vi "Control_Create.vi"(0 "reference in":refnum<class "Control.lvclass">, 1 "Object Attributes":T1, 2 "Control Attributes":T3, 5 "error in (no error)":errorcluster) -> (14 "reference out":refnum<class "Control.lvclass">, 19 "error out":errorcluster)   [LabVIEW 2014, in "Control.lvclass"]
uses:
  Control.lvclass
  Attributes.ctl
  Text_class/Text.lvclass
  <vilib>/picture/picture.llb/imagedata.ctl
  Object_class/Attributes.ctl
  Object_class/Coordinates.ctl
  Object_class/Object.lvclass
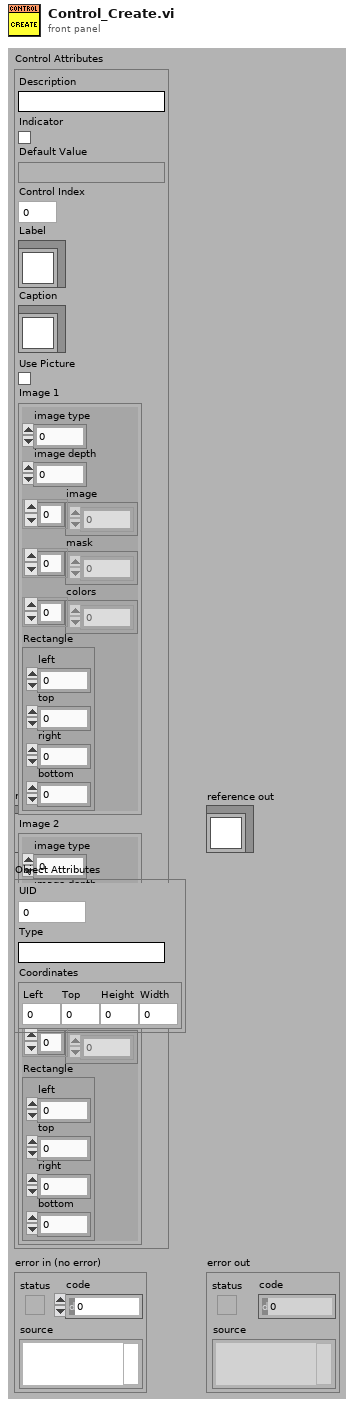
[diagram p1: front panel]
types:
  T1 = typedef "Object.lvclass/Attributes.ctl" = cluster{"UID":i32, "Type":string, "Coordinates":T2}
  T2 = typedef "Object.lvclass/Coordinates.ctl" = cluster{"Left":i32, "Top":i32, "Height":u32, "Width":u32}
  T3 = typedef "Control.lvclass/Attributes.ctl" = cluster{"Description":string, "Indicator":bool, "Default Value":variant, "Control Index":i32, "Label":refnum<class "Text.lvclass">, "Caption":refnum<class "Text.lvclass">, "Use Picture":bool, "Image 1":T4, "Image 2":T4}
  T4 = typedef "imagedata.ctl" = cluster{"image type":i32, "image depth":i32, "image":u8[], "mask":u8[], "colors":u32[], "Rectangle":cluster{"left":i16, "top":i16, "right":i16, "bottom":i16}}
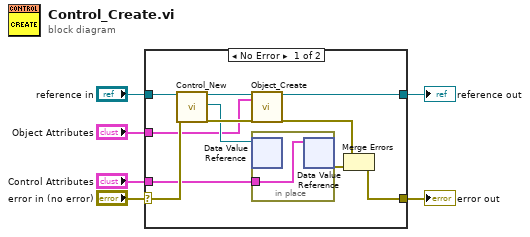
[diagram p0: block diagram]
diagram:
  n1 = case shown="No Error" "error in (no error)" {
    selector: "error in (no error)" -> [w16 w20]
    tunnel: [w14 w20] -> w5
    tunnel: "reference in" -> [w17 w19]
    tunnel: [w11 w19] -> w3
    tunnel: "Object Attributes" -> [w9 _]
    tunnel: "Control Attributes" -> [w8 _]
    frame No Error {
      n2 = call "Control_New.vi"("reference in"=w17, "error in (no error)"=w16) -> ("reference out"=w13:refnum<class "Control.lvclass">, "DVRRefOut"=w10:refnum<data-value>, "error out"=w12:errorcluster)  [unwired: 14 in, 1 out]
      n3 = call "Object_Create.vi"("reference in"=w13, "Object Attributes"=w9, "error in (no error)"=w12) -> ("reference out"=w11:refnum<class "Control.lvclass">, "error out"=w7:errorcluster)  [unwired: 15 in]
      n4 = in-place {
        in-place-border: w8 -> [w18]
        n5 = in-place-dvr #1(w10) -> ()  [unwired: 2 out]
        n6 = in-place-dvr #1(w18) -> (w15:errorcluster)  [unwired: 1 out]
      }
      n7 = Merge Errors(w7, w15) -> (w14:errorcluster)
    }
    frame Error {
    }
  }
  "error out" <- w5
  "reference out" <- w3
